vi "Check if at destination.vi"(8 "error in (no error)":errorcluster, 11 "StageSPIM in":refnum<class "StageSPIM.lvclass">) -> (0 "error out":errorcluster, 1 "focus at destination?":bool, 2 "at destination? (all but focus)":bool, 3 "StageSPIM out":refnum<class "StageSPIM.lvclass">)   [LabVIEW 2012, in "StageSPIM.lvclass"]
uses:
  StageSPIM.lvclass
  StageSPIM.lvclass/StageSPIM.ctl
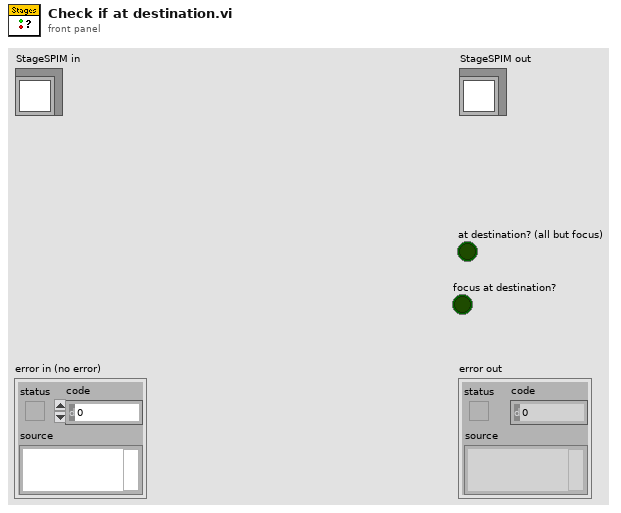
[diagram p1: front panel]
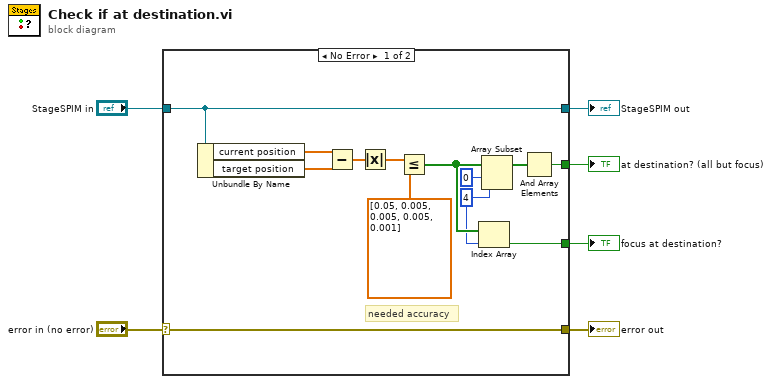
[diagram p0: block diagram]
diagram:
  n1 = case shown="No Error" "error in (no error)" {
    selector: "error in (no error)" -> [w19 w21]
    tunnel: [w19 w21] -> w5
    tunnel: [w18 w20] -> w3
    tunnel: "StageSPIM in" -> [w18 w20]
    tunnel: [w12 _] -> w2
    tunnel: [w7 _] -> w1
    frame No Error {
      w8 = 4 ("length")
      # "needed accuracy"
      n2 = Unbundle By Name(w18) -> ("current position"=w17:dbl[], "target position"=w16:dbl[])
      n3 = Subtract(x=w17, y=w16) -> (x-y=w15:dbl[])
      n4 = Absolute Value(x=w15) -> (abs(x)=w14:dbl[])
      n5 = Less Or Equal?(x=w14, y=dbl[] [0.05, 0.005, 0.005, 0.005, 0.001]) -> (x <= y?=w10:bool[])
      n6 = Index Array(array=w10, index=w8) -> (element=w7:bool)
      n7 = Array Subset(array=w10, index=0, length=w8) -> (w9:bool[])
      n8 = And Array Elements(Boolean array=w9) -> (logical AND=w12:bool)
    }
    frame Error {
    }
  }
  "error out" <- w5
  "StageSPIM out" <- w3
  "at destination? (all but focus)" <- w2
  "focus at destination?" <- w1
